vi "Sensor Poka Yoka.vi"(9 "Digital input":bool[](array[boolean])) -> (2 "Pokayoka":T1)   [LabVIEW 2015]
panel:
  in  "Pokayoka 2":T1
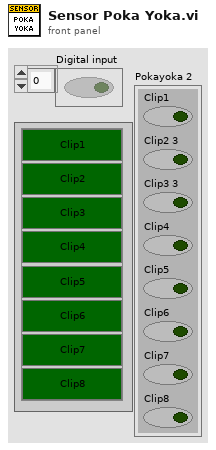
[diagram p1: front panel]
types:
  T1 = cluster{"Clip1":bool, "Clip2 3":bool, "Clip3 3":bool, "Clip4":bool, "Clip5":bool, "Clip6":bool, "Clip7":bool, "Clip8":bool}
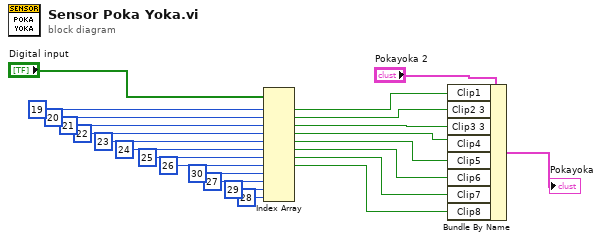
[diagram p0: block diagram]
diagram:
  n1 = Index Array(array="Digital input", index #1=19 ("index"), index #2=20 ("index"), index #3=21 ("index"), index #4=22 ("index"), index #5=23 ("index"), index #6=24 ("index"), index #7=25 ("index"), index #8=26 ("index"), index #9=30 ("index"), index #10=27 ("index"), index #11=29 ("index"), index #12=28 ("index")) -> (element #1=w8:bool, element #2=w9:bool, element #3=w10:bool, element #4=w11:bool, element #5=w12:bool, element #6=w13:bool, element #7=w14:bool, element #8=w15:bool)  [unwired: 4 out]
  n2 = Bundle By Name(cluster="Pokayoka 2", "Clip1"=w8, "Clip2 3"=w9, "Clip3 3"=w10, "Clip4"=w11, "Clip5"=w12, "Clip6"=w13, "Clip7"=w14, "Clip8"=w15) -> (→"Pokayoka":T1)
